vi "close.vi"(8 "error in (no error)":errorcluster, 11 "Lakeshore 325 in":refnum<class "Lakeshore 325.lvclass">) -> (0 "error out":errorcluster, 3 "Lakeshore 325 out":refnum<class "Lakeshore 325.lvclass">)   [LabVIEW 2022 SP3, in "Lakeshore 325.lvclass"]
uses:
  Lakeshore 325.lvclass
  Lakeshore 325.lvclass/Lakeshore 325.ctl
  Temp Control.lvclass
  <instrlib>/Lake Shore 325/Lake Shore 325.lvlib
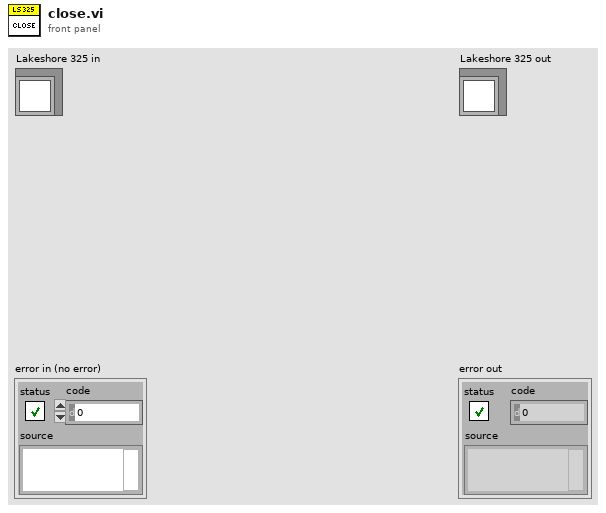
[diagram p1: front panel]
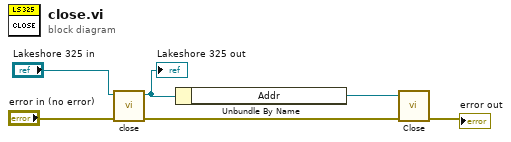
[diagram p0: block diagram]
diagram:
  n1 = call-parent <instrlib>:"close.vi"("error in (no error)"="error in (no error)", "Temp Control in"="Lakeshore 325 in") -> ("error out"=w2:errorcluster, "Temp Control out"=w4:refnum<class "Lakeshore 325.lvclass">)  [unwired: 8 in]
  "Lakeshore 325 out" <- w4
  n2 = Unbundle By Name(w4) -> ("Addr"=w3:refnum<visa-resource-name>)
  n3 = call <instrlib>:"Close.vi"("error in (no error)"=w2, "VISA resource name"=w3) -> ("error out"=→"error out":errorcluster)  [unwired: 9 in]
